vi "XYStage.ConvertCoordinates.vi"(8 "error in (no error)":errorcluster, 9 "Counts":T1, 10 "Real Units Coords":T2, 11 "XYStage in":refnum<class "XYStage.lvclass">) -> (0 "error out":errorcluster, 1 "Real Units Coords out":T2, 2 "Counts out":T1, 3 "XYStage out":refnum<class "XYStage.lvclass">)   [LabVIEW 2015, in "XYStage.lvclass"]
uses:
  XYStage.lvclass
  Typedefs/(real)Coords--Cluster.ctl
  Typedefs/(counts)Coords--Cluster.ctl
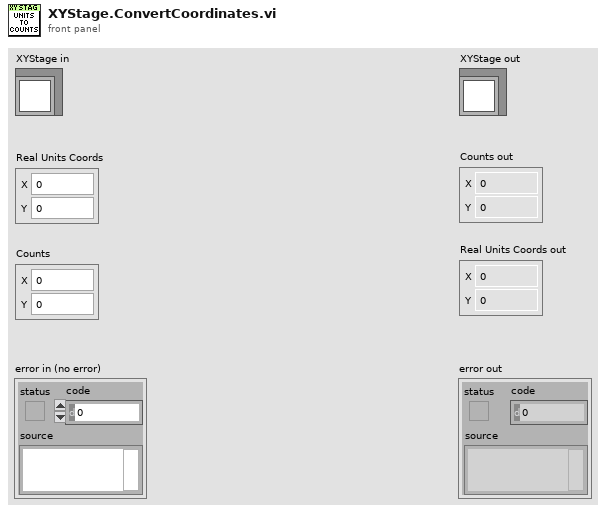
[diagram p1: front panel]
types:
  T1 = typedef "XYStage.lvclass/(counts)Coords--Cluster.ctl" = cluster{"X":i32, "Y":i32}
  T2 = typedef "XYStage.lvclass/(real)Coords--Cluster.ctl" = cluster{"X":dbl, "Y":dbl}
  T3 = typedef "XYStage.lvclass/Configuration--Cluster.ctl" = cluster{"Real-World Units":string, "Counts per Unit":dbl}
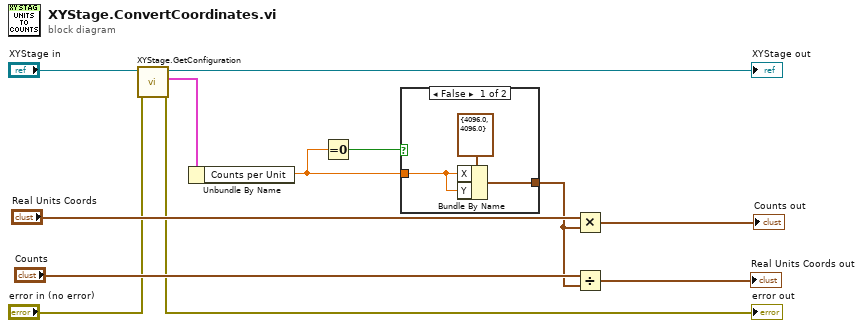
[diagram p0: block diagram]
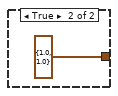
[diagram p2: hidden frame]
diagram:
  n1 = call "XYStage.GetConfiguration.vi"("error in (no error)"="error in (no error)", "XYStage"="XYStage in") -> ("error out"=→"error out":errorcluster, "Configuration"=w3:T3, "XYStage out"=→"XYStage out":refnum<class "XYStage.lvclass">)  [unwired: 7 in]
  n2 = Unbundle By Name(w3) -> ("Counts per Unit"=w2:dbl)
  n3 = Equal To 0?(x=w2) -> (x = 0?=w1:bool)
  n4 = case shown="False" w1 {
    tunnel: [w14 T2 {"X"=1.0, "Y"=1.0} ("y")] -> w4
    tunnel: w2 -> [w13 _]
    frame False {
      n5 = Bundle By Name(cluster=T2 {"X"=4096.0, "Y"=4096.0} ("y"), "X"=w13, "Y"=w13) -> (w14:T2)
    }
    frame True {
    }
  }
  n6 = Multiply(x="Real Units Coords", y=w4) -> (x*y=→"Counts out":T2)
  n7 = Divide(x="Counts", y=w4) -> (x/y=→"Real Units Coords out":T2)
